vi "Configure Horizontal.vi"(8 "error in":errorcluster, 11 "object in":refnum<class "Fetch Waveforms CFG.lvclass">) -> (0 "error out":errorcluster, 3 "object out":refnum<class "Fetch Waveforms CFG.lvclass">)   [LabVIEW 2023, in "Scope Simulated CFGs.lvlib" / "Fetch Waveforms CFG.lvclass"]
uses:
  Fetch Waveforms CFG.lvclass
  Fetch Waveforms CFG.lvclass/Fetch Waveforms CFG.ctl
  <vilib>/Utility/error.llb/Error Cluster From Error Code.vi
  <vilib>/ErrorRing/Error Ring.xnode
  Configuration JSON Base/CFG JSON Base.lvclass
  2e7921dc-a2d8-456a-8bcd-efe2ea717c44.vi
panel:
  out "Data":T1
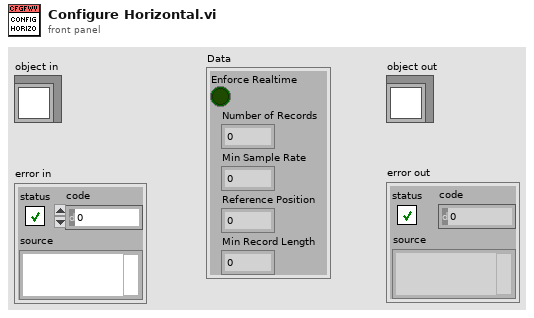
[diagram p1: front panel]
types:
  T1 = cluster{"Enforce Realtime":bool, "Number of Records":i32, "Min Sample Rate":dbl, "Reference Position":dbl, "Min Record Length":i32}
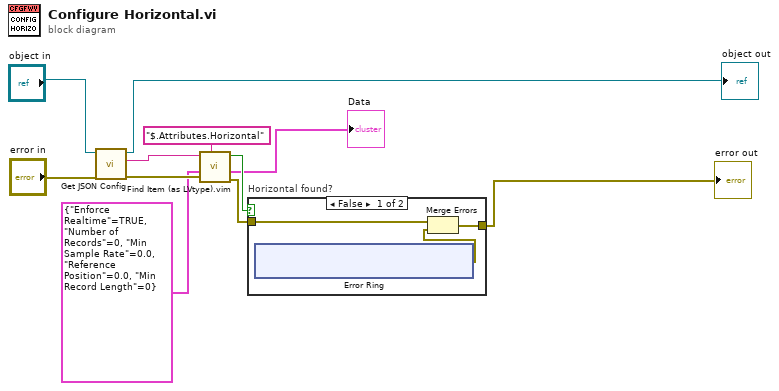
[diagram p0: block diagram]
diagram:
  n1 = call "Get JSON Config.vi"("error in (no error)"="error in", "CFG Base in"="object in") -> ("error out"=w9:errorcluster, "<JSON>Config>"=w8:string, "CFG Base out"=→"object out":refnum<class "Fetch Waveforms CFG.lvclass">)  [unwired: 7 in]
  n2 = call "Find Item (as LVtype).vim"("$Path or Item Name"="$.Attributes.Horizontal", "error in (no error)"=w9, "Data Type and Default Value"=T1 {"Enforce Realtime"=TRUE, "Number of Records"=0, "Min Sample Rate"=0.0, "Reference Position"=0.0, "Min Record Length"=0}, "JSON"=w8) -> ("error out"=w6:errorcluster, "Data"=→"Data":T1, "Found"=w5:bool)  [unwired: 4 in, 1 out]
  n3 = case "Horizontal found?" shown="False" w5 {
    tunnel: [w14 w20] -> w2
    tunnel: w6 -> [w12 w20]
    frame False {
      n4 = xnode "Error Ring"() -> ("error out"=w13:errorcluster)
      n5 = Merge Errors(w12, w13) -> (w14:errorcluster)
    }
    frame True {
    }
  }
  "error out" <- w2
